vi "Interpolation_SortedX_Y.vi"(1 "Y Data":dbl[](array[numeric]), 2 "X Data (sorted)":dbl[](array[numeric]), 3 "Target X (threshold)":dbl) -> (0 "Interpolated Results":dbl)   [LabVIEW 2017]
doc: "Interpolate. Enter Target X (threshold) value which should be a value between sorted X data array values. It will find the corresponding Y data value."
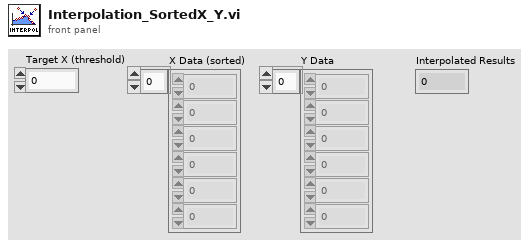
[diagram p1: front panel]
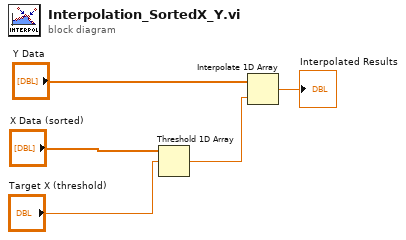
[diagram p0: block diagram]
diagram:
  n1 = Threshold 1D Array(2:"Target X (threshold)", 3:"X Data (sorted)") -> (0:w5:dbl)  [unwired: 1 in]
  n2 = Interpolate 1D Array(1:w5, 2:"Y Data") -> (0:→"Interpolated Results":dbl)
